vi "Send Immediate Return Round Trip Message.vi"(8 "error in (no error)":errorcluster, 10 "Return Enqueuer (Self)":refnum<class "Message Enqueuer.lvclass">, 11 "Message Enqueuer (Remote Actor)":refnum<class "Message Enqueuer.lvclass">) -> (0 "error out":errorcluster, 2 "Leak The Round-Trip Message For Test":refnum<class "ImmediateReturnRoundTripMessage.lvclass">, 3 "Message Enqueuer out":refnum<class "Message Enqueuer.lvclass">)   [LabVIEW 2017, in "ImmediateReturnRoundTripMessage.lvclass"]
uses:
  ImmediateReturnRoundTripMessage.lvclass
  <vilib>/ActorFramework/Message Enqueuer/Message Enqueuer.lvclass
  C:/Git/composed-af-messages/Source/AddressedMessage/RoundTripMessage.lvclass
  C:/Program Files (x86)/National Instruments/LabVIEW 2017/vi.lib/ActorFramework/Message/Message.lvclass
  Source/RoundTripMessage/RoundTripMessage.lvclass/RoundTripMessage.ctl
  <vilib>/ActorFramework/Message Enqueuer/Message Enqueuer.lvclass/Message Enqueuer.ctl
  <vilib>/ActorFramework/Message Priority Queue/Priority Enqueue.vi
  Source/RoundTripMessage/RoundTripMessage.lvclass
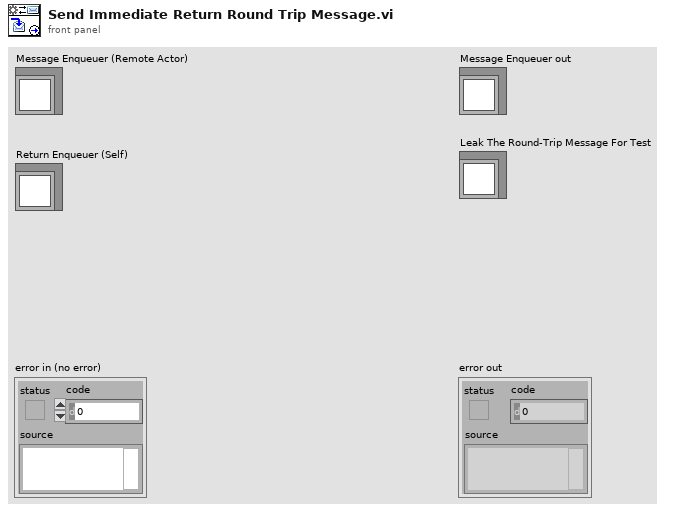
[diagram p1: front panel]
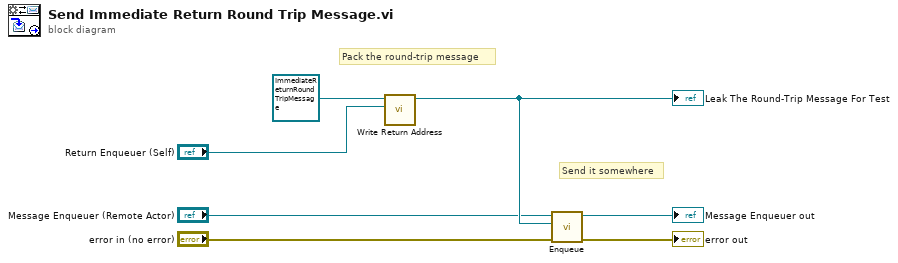
[diagram p0: block diagram]
diagram:
  # "Send it somewhere"
  # "Pack the round-trip message"
  n1 = call "Write Return Address.vi"("Return Enqueuer"="Return Enqueuer (Self)", "RoundTripMessage In"=refnum<class "ImmediateReturnRoundTripMessage.lvclass"> refnum ("ImmediateReturnRoundTripMessage out")) -> ("RoundTripMessage Out"=w4:refnum<class "ImmediateReturnRoundTripMessage.lvclass">)  [unwired: 9 in]
  "Leak The Round-Trip Message For Test" <- w4
  n2 = call <vilib>:"Enqueue.vi"("error in (no error)"="error in (no error)", "Message"=w4, "Message Enqueuer in"="Message Enqueuer (Remote Actor)") -> ("error out"=→"error out":errorcluster, "Message Enqueuer out"=→"Message Enqueuer out":refnum<class "Message Enqueuer.lvclass">)  [unwired: 7 in]
